vi "WriteTYPE_NAME.vi"(8 "error in (no error)":errorcluster, 10 "TYPE_NAME":string, 11 "object in":refnum<class "SetInputValue.lvclass">) -> (0 "error out":errorcluster, 3 "object out":refnum<class "SetInputValue.lvclass">)   [LabVIEW 2017, in "SetInputValue.lvclass"]
uses:
  SetInputValue.lvclass
  SetInputValue.lvclass/SetInputValue.ctl
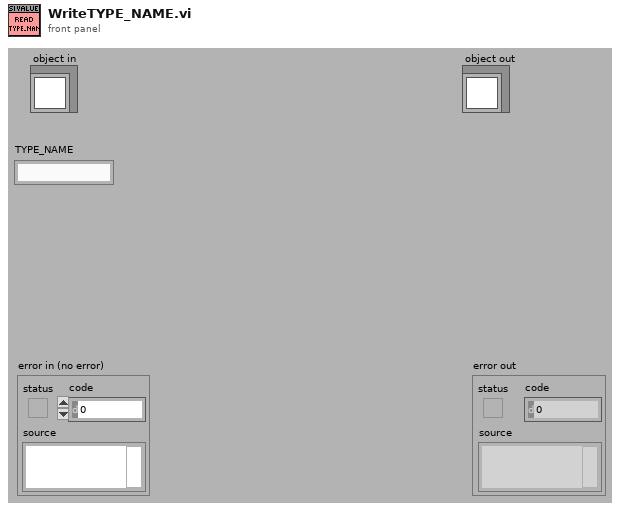
[diagram p1: front panel]
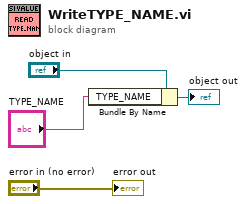
[diagram p0: block diagram]
diagram:
  n1 = Bundle By Name(cluster="object in", "TYPE_NAME"="TYPE_NAME") -> (→"object out":refnum<class "SetInputValue.lvclass">)
  "error out" <- "error in (no error)"
